vi "Simple calculator.vi"() -> ()   [LabVIEW 2015]
panel:
  out "Result":dbl
  in  "Operation":string(combo)
  in  "Y input":dbl
  in  "X input":dbl
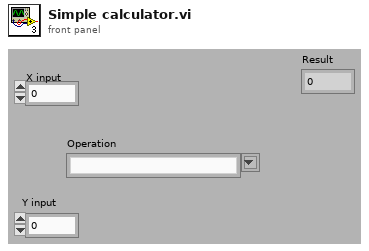
[diagram p1: front panel]
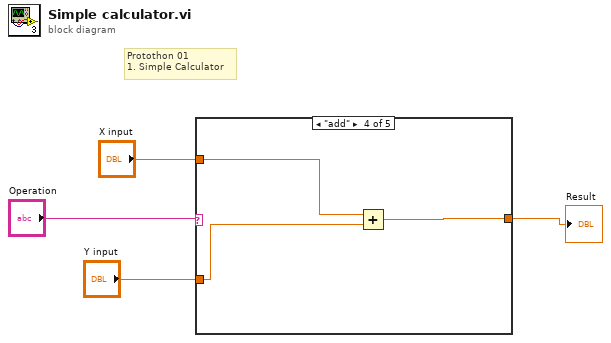
[diagram p0: block diagram]
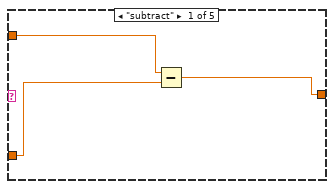
[diagram p2: hidden frame]
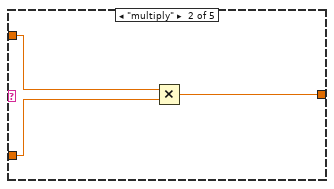
[diagram p3: hidden frame]
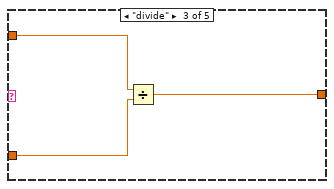
[diagram p4: hidden frame]
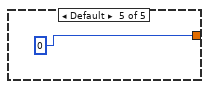
[diagram p5: hidden frame]
diagram:
  # "Protothon 01\n1. Simple Calculator"
  n1 = case shown="\"add\"" "Operation" {
    tunnel: "Y input" -> [w6 w9 w13 w15 _]
    tunnel: "X input" -> [w7 w10 w12 w16 _]
    tunnel: [w5 w8 w11 w14 0] -> w1
    frame "subtract" {
      n2 = Subtract(x=w7, y=w6) -> (x-y=w5:dbl)
    }
    frame "multiply" {
      n3 = Multiply(x=w10, y=w9) -> (x*y=w8:dbl)
    }
    frame "divide" {
      n4 = Divide(x=w12, y=w13) -> (x/y=w11:dbl)
    }
    frame "add" {
      n5 = Add(x=w16, y=w15) -> (x+y=w14:dbl)
    }
    frame Default {
    }
  }
  "Result" <- w1
